vi "Blob ReadInfo.vi"(8 "error in (no error)":errorcluster, 11 "Blob in":refnum<class "Blob.lvclass">) -> (0 "error out":errorcluster, 2 "BlobInfo":T1, 3 "Blob out":refnum<class "Blob.lvclass">)   [LabVIEW 2020, in "OpenLvVision_OpenCv.lvlib" / "Blob.lvclass"]
doc: "Return the size and type of the blob."
uses:
  Blob.lvclass
  C:/Users/lukas/Downloads/OpenLvVision_OpenCv/SourceCode/LabView/OpenLvVision_OpenCv/_LvHelpers/EdvrObject/EdvrObject.lvclass
  TypeDef/BlobInfo.ctl
  TypeDef/NchwType.ctl
  _LvHelpers/EdvrObject/EdvrObject.lvclass/EdvrObject.ctl
  OpenLvVision_OpenCv.lvlib
  _LvHelpers/EdvrObject/EdvrObject.lvclass
  Dlls/OlvOpenCvWrapper.dll
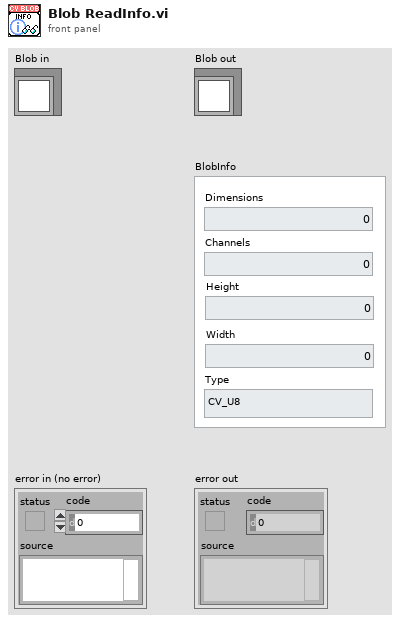
[diagram p1: front panel]
types:
  T1 = typedef "OpenLvVision_OpenCv.lvlib/BlobInfo.ctl" = cluster{"Dimensions":i32, "Channels":i32, "Height":i32, "Width":i32, "Type":T2}
  T2 = typedef "OpenLvVision_OpenCv.lvlib/NchwType.ctl" = enum16{"CV_U8", "CV_8S", "CV_16U", "CV_16S", "CV_32S", "CV_32F", "CV_64F", "CV_16F"}
  T3 = typedef "OpenLvVision_OpenCv.lvlib/EdvrObject.lvclass/Edvr.ctl" = refnum<data-value>
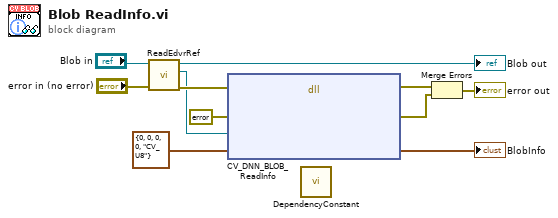
[diagram p0: block diagram]
diagram:
  n1 = call "ReadEdvrRef.vi"("error in (no error)"="error in (no error)", "EdvrObject in"="Blob in") -> ("error out"=w9:errorcluster, "Edvr"=w8:T3, "EdvrObject out"=→"Blob out":refnum<class "Blob.lvclass">)  [unwired: 7 in]
  n2 = dll-call lib="C:/Users/lukas/Downloads/OpenLvVision_OpenCv/SourceCode/LabView/OpenLvVision_OpenCv/Dlls/OlvOpenCvWrapper.dll" fn="CV_DNN_BLOB_ReadInfo"(error in=w9, "Error"=errorcluster {"status"=FALSE, "code"=0, "source"=""} ("error out"), "edvrRef"=w8, "Shape"=T1 {"Dimensions"=0, "Channels"=0, "Height"=0, "Width"=0, "Type"=enum."CV_U8"} ("BlobInfo")) -> (error out=w6:errorcluster, "Error"=w5:errorcluster, "Shape"=→"BlobInfo":T1)  [unwired: 4 in, 1 out]
  n3 = call "DependencyConstant.vi"() -> ()  [unwired: 12 in]
  n4 = Merge Errors(w6, w5) -> (→"error out":errorcluster)
